vi "LVClass_CorrectionDataManager SetActuatorPrefs.vi"(0 "CorrectionDataManager in":refnum<class "CorrectionDataManager.lvclass">, 5 "Index of actuator":dbl, 7 "Actuator state":T1, 11 "error in (no error)":errorcluster) -> (4 "CorrectionDataManager out":refnum<class "CorrectionDataManager.lvclass">, 8 "New data Need":bool, 15 "error out":errorcluster)   [LabVIEW 2020, in "CorrectionDataManager.lvclass"]
doc: "Preferences setter for one wavefront corrector actuator. .\n\n<B>corrdata_managerIn</B> : CorrDataManager object.\n<B>corrdata_managerOut</B> : CorrDataManager object.\n<B>actuator_index</B> : Index of the actuator.\n<B>min</B> : WavefrontCorrector actuator preferences : lowest command value.\n<B>max</B> : WavefrontCorrector actuator preferences : highest command value.\n<B>validity</B> : WavefrontCorrector actuator preferences : status.\n<B>fixed_value</B> : WavefrontCorrector actuator preferences : fixed positions.\n<B>new_data_needed</B> : if true, indicates that interaction matrix has been erased."
uses:
  CorrectionDataManager.lvclass
  Wavefront Corrector states - ONE.ctl
  CorrectionDataManager.lvclass/CorrectionDataManager.ctl
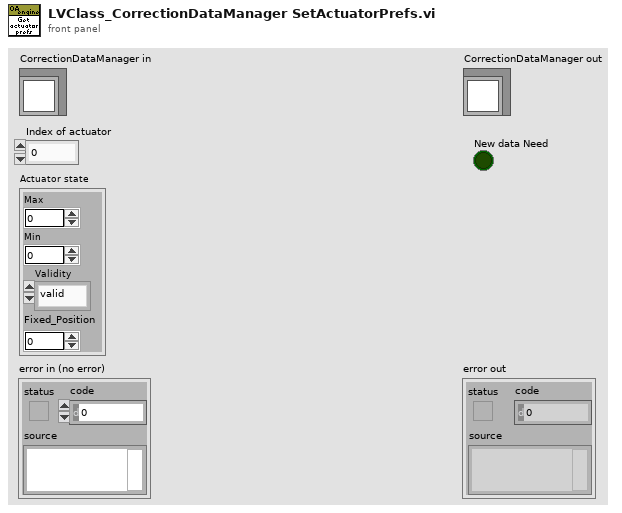
[diagram p1: front panel]
types:
  T1 = typedef "Wavefront Corrector states - ONE.ctl" = cluster{"Max":sgl, "Min":sgl, "Validity":enum16{"valid", "fixed", "invalid"}, "Fixed_Position":sgl}
  T2 = typedef "ClassID.ctl" = i64
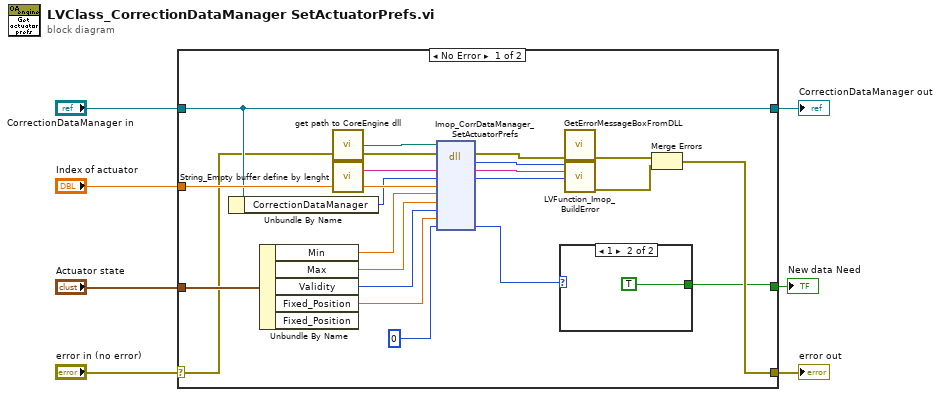
[diagram p0: block diagram]
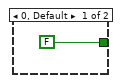
[diagram p2: hidden frame]
diagram:
  n1 = case shown="No Error" "error in (no error)" {
    selector: "error in (no error)" -> [w13 w32]
    tunnel: [w12 w32] -> w6
    tunnel: [w20 w31] -> w4
    tunnel: "CorrectionDataManager in" -> [w20 w31]
    tunnel: "Index of actuator" -> [w21 _]
    tunnel: "Actuator state" -> [w18 _]
    tunnel: [w9 _] -> w1
    frame No Error {
      n2 = Unbundle By Name(w20) -> ("CorrectionDataManager"=w19:T2)
      n3 = Unbundle By Name(w18) -> ("Min"=w17:sgl, "Max"=w16:sgl, "Validity"=w15:enum16{"valid", "fixed", "invalid"}, "Fixed_Position"=w14:sgl)  [unwired: 1 out]
      n4 = call "get path to CoreEngine dll.vi"() -> ("path to wavekit library"=w26:path)  [unwired: 14 in, 1 out]
      n5 = call "String_Empty buffer define by lenght.vi"() -> ("Empty buffer"=w25:string)  [unwired: 1 in]
      n6 = dll-call lib="D:/FLE/0.Code/CoreEngine4_Suite/LV2011_interface/DLLs/c_interface_vc100.dll" fn="Imop_CorrDataManager_SetActuatorPrefs"(path in=w26, error in=w13, "Message"=w25, "CorrectionDataManager"=w19, "Actuator index"=w21, "Min"=w17, "Max"=w16, "Validity"=w15, "Fixed position"=w14, "New data needed"=u8 0) -> (error out=w24:errorcluster, "return type"=w23:i32, "Message"=w22:string, "CorrectionDataManager"=w8:i64, "New data needed"=w10:u8)  [unwired: 6 in, 1 out]
      n7 = case shown="1" w10 {
        tunnel: [FALSE TRUE] -> w9
        frame 0, Default {
        }
        frame 1 {
        }
      }
      n8 = call "GetErrorMessageBoxFromDLL.vi"("error IN"=w24) -> ("error OUT"=w28:errorcluster)  [unwired: 10 in]
      n9 = call "LVFunction_Imop_BuildError.vi"("code"=w23, "String to Prepend to source (\"\")"=w22, "Adresse"=w8) -> ("error out"=w27:errorcluster)  [unwired: 12 in]
      n10 = Merge Errors(w28, w27) -> (w12:errorcluster)
    }
    frame Error {
    }
  }
  "error out" <- w6
  "CorrectionDataManager out" <- w4
  "New data Need" <- w1
